vi "SetParentTag.vi"(8 "error in (no error)":errorcluster, 10 "Parent Tag":string, 11 "ClassDataTree in":refnum<class "ClassDataTree.lvclass">) -> (0 "error out":errorcluster, 3 "ClassDataTree out":refnum<class "ClassDataTree.lvclass">)   [LabVIEW 2010, in "ClassDataTree.lvclass"]
uses:
  ClassDataTree.lvclass
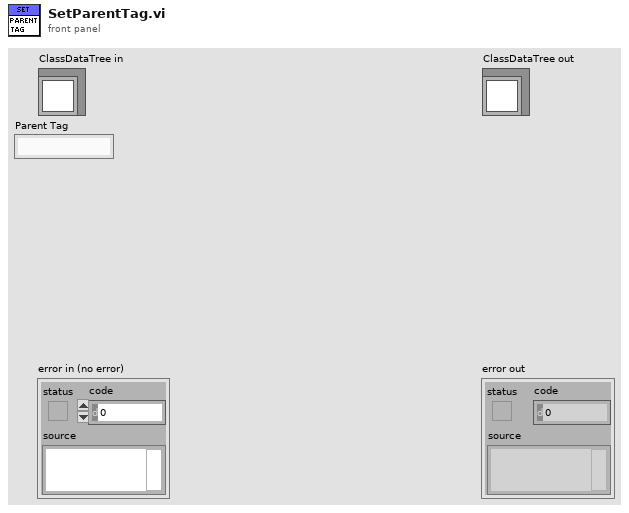
[diagram p1: front panel]
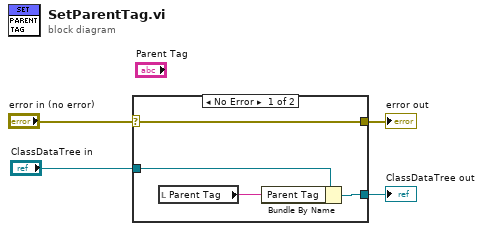
[diagram p0: block diagram]
diagram:
  n1 = case shown="No Error" "error in (no error)" {
    selector: "error in (no error)" -> [w8 w10]
    tunnel: [w8 w10] -> w3
    tunnel: [w6 w9] -> w1
    tunnel: "ClassDataTree in" -> [w7 w9]
    frame No Error {
      n2 = local read "Parent Tag"() -> (w5:string)
      n3 = Bundle By Name(cluster=w7, "Parent Tag"=w5) -> (w6:refnum<class "ClassDataTree.lvclass">)
    }
    frame Error {
    }
  }
  "error out" <- w3
  "ClassDataTree out" <- w1
